vi "p33_1_oa2r.vi"() -> ()   [LabVIEW 2013]
panel:
  out "transformation matrix":picture
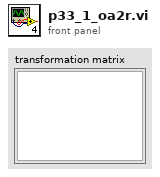
[diagram p1: front panel]
types:
  T1 = typedef "NI_Matrix.lvlib/RealMatrix.ctl" = dbl[][]
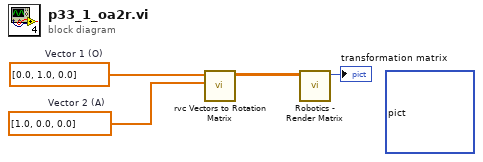
[diagram p0: block diagram]
diagram:
  (unwired) picture bytes[500] ("transformation matrix")
  w2 = dbl[] [1.0, 0.0, 0.0]  # Vector 2 (A)
  w3 = dbl[] [0.0, 1.0, 0.0]  # Vector 1 (O)
  n1 = call "rvc Vectors to Rotation Matrix.vi"("Vector 2 (A)"=w2, "Vector 1 (O)"=w3) -> ("rotation matrix"=w1:T1)  [unwired: 9 in]
  n2 = call "Robotics - Render Matrix.vi"("A"=w1) -> ("picture out"=→"transformation matrix":picture)  [unwired: 10 in]
